vi "单次收发模式.vi"() -> ()   [LabVIEW 2017]
uses:
  <vilib>/Instr/_visa.llb/VISA Configure Serial Port (Instr).vi
  <vilib>/ptbypt/NI_PtbyPt.lvlib
panel:
  out "波形图表":cluster{dbl, dbl, dbl}(graph)
  out "Fz":dbl
  out "Fy":dbl
  out "Fx":dbl
  out "连接的字符串":string
  out "频率/Hz":dbl
  out "relative seconds":dbl caption="相对秒钟" format="%_19f"
  in  "置零":bool
  in  "停止":bool
  in  "传感器串口号":refnum<visa-resource-name>
  out "读取缓冲区":string
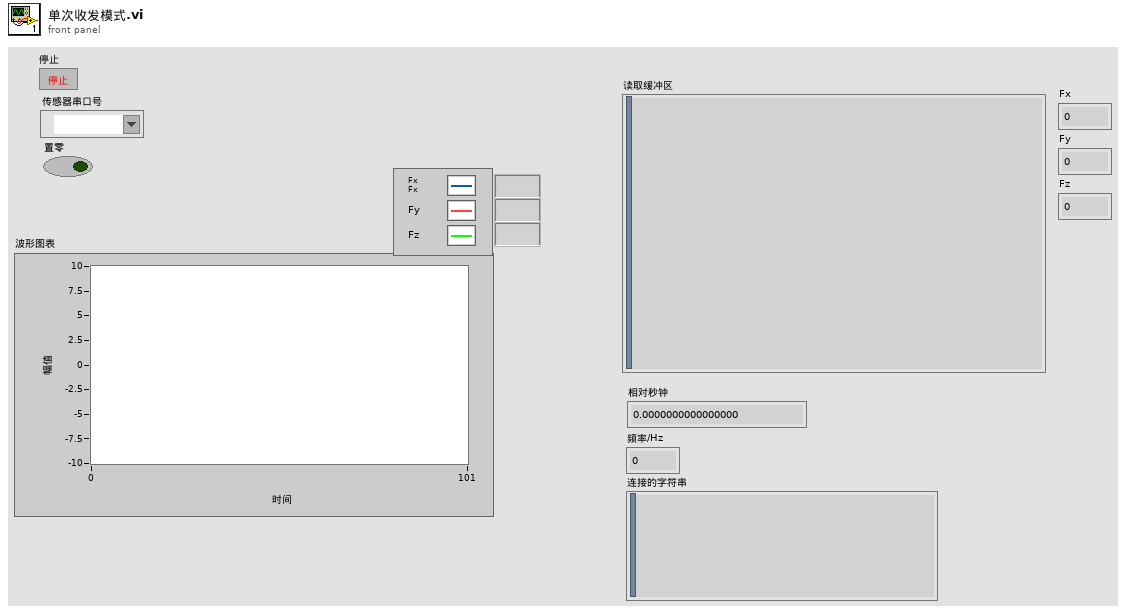
[diagram p1: front panel]
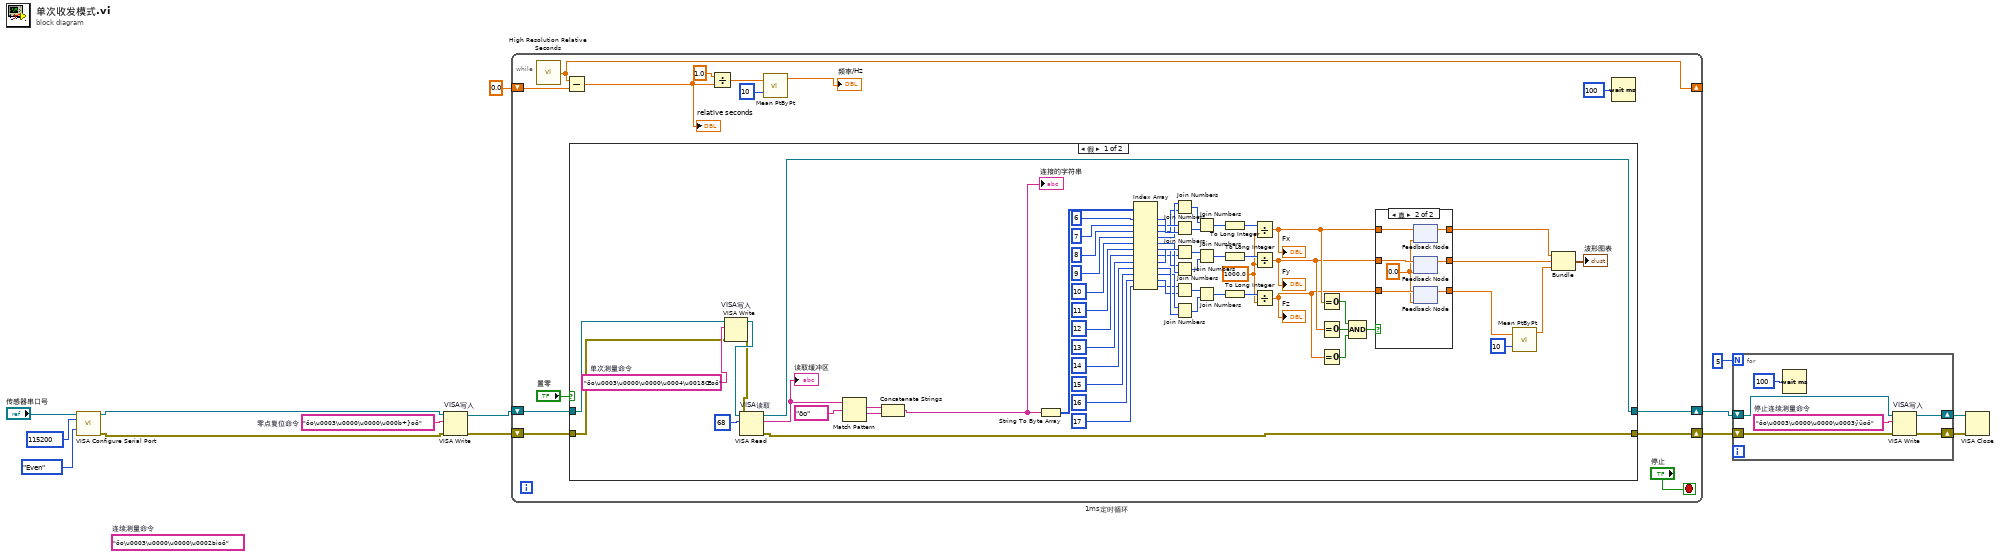
[diagram p0: block diagram]
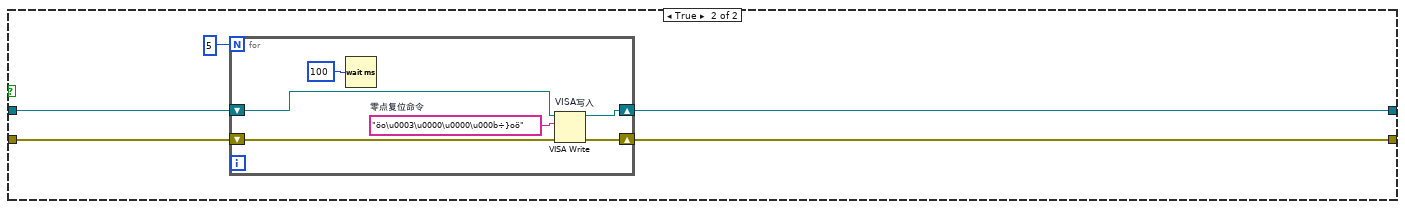
[diagram p3: hidden frame]
diagram:
  w2 = "öo\u0003\u0000\u0000\u000b÷}oö"  # 零点复位命令
  (unwired) "öo\u0003\u0000\u0000\u0002Þìoö"  # 连续测量命令
  n1 = call-poly "VISA Configure Serial Port"("VISA resource name"="传感器串口号", "baud rate (9600)"=u32 115200, "parity (0:none)"=enum16{"None", "Odd", "Even", "Mark", "Space"}."Even") -> ("VISA resource name out"=w12:refnum<visa-resource-name>, "error out"=w11:errorcluster)  [unwired: 11 in]
  n2 = VISA Write "VISA写入"(VISA resource name=w12, write buffer=w2, error in (no error)=w11) -> (VISA resource name out=w4:refnum<visa-resource-name>, error out=w3:errorcluster)  [unwired: 1 out]
  n3 = while "1ms定时循环" {
    shift-right: [w26] -> w9
    shift-left: w4 -> [w28]
    shift-right: [w25] -> w8
    shift-left: w3 -> [w27]
    shift-right: [w22] -> _
    shift-left: 0.0 ("relative seconds") -> [w21]
    stop <- "停止" stop-if-true
    n4 = call <vilib>:"High Resolution Relative Seconds.vi"() -> ("relative seconds"=w22:dbl)
    n5 = Subtract(x=w22, y=w21) -> (x-y=w20:dbl)
    "relative seconds" <- w20
    n6 = case shown="假" "置零" {
      tunnel: w28 -> [w33 w105]
      tunnel: w27 -> [w32 w107]
      tunnel: [w91 w104] -> w26
      tunnel: [w90 w106] -> w25
      frame False {
        w34 = "öo\u0003\u0000\u0000\u0004\u0018Œoö"  # 单次测量命令
        w59 = 1000.0
        n7 = VISA Write "VISA写入"(VISA resource name=w33, write buffer=w34, error in (no error)=w32) -> (VISA resource name out=w31:refnum<visa-resource-name>, error out=w30:errorcluster)  [unwired: 1 out]
        n8 = VISA Read "VISA读取"(VISA resource name=w31, byte count=u32 68 ("字节总数"), error in (no error)=w30) -> (VISA resource name out=w91:refnum<visa-resource-name>, read buffer=w89:string, error out=w90:errorcluster)  [unwired: 1 out]
        "读取缓冲区" <- w89
        n9 = Match Pattern(string=w89, regular expression="öo" ("正则表达式")) -> (match substring=w85:string, after substring=w84:string)  [unwired: 1 in, 2 out]
        n10 = Concatenate Strings(w85, w84) -> (w29:string)
        "连接的字符串" <- w29
        n11 = String To Byte Array(string=w29) -> (unsigned byte array=w87:u8[])
        n12 = Index Array(array=w87, index #1=6 ("索引"), index #2=7 ("索引"), index #3=8 ("索引"), index #4=9 ("索引"), index #5=10 ("索引"), index #6=11 ("索引"), index #7=12 ("索引"), index #8=13 ("索引"), index #9=14 ("索引"), index #10=15 ("索引"), index #11=16 ("索引"), index #12=17 ("索引")) -> (element #1=w83:u8, element #2=w82:u8, element #3=w80:u8, element #4=w81:u8, element #5=w73:u8, element #6=w72:u8, element #7=w71:u8, element #8=w74:u8, element #9=w66:u8, element #10=w65:u8, element #11=w64:u8, element #12=w63:u8)
        n13 = Join Numbers(hi=w81, lo=w80) -> ((hi.lo)=w78:u16)
        n14 = Join Numbers(hi=w82, lo=w83) -> ((hi.lo)=w79:u16)
        n15 = Join Numbers(hi=w74, lo=w71) -> ((hi.lo)=w76:u16)
        n16 = Join Numbers(hi=w72, lo=w73) -> ((hi.lo)=w75:u16)
        n17 = Join Numbers(hi=w63, lo=w64) -> ((hi.lo)=w67:u16)
        n18 = Join Numbers(hi=w65, lo=w66) -> ((hi.lo)=w68:u16)
        n19 = Join Numbers(hi=w78, lo=w79) -> ((hi.lo)=w77:u32)
        n20 = Join Numbers(hi=w76, lo=w75) -> ((hi.lo)=w70:u32)
        n21 = Join Numbers(hi=w67, lo=w68) -> ((hi.lo)=w69:u32)
        n22 = To Long Integer(number=w77) -> (32bit integer=w62:i32)
        n23 = To Long Integer(number=w70) -> (32bit integer=w60:i32)
        n24 = To Long Integer(number=w69) -> (32bit integer=w61:i32)
        n25 = Divide(x=w62, y=w59) -> (x/y=w42:dbl)
        "Fx" <- w42
        n26 = Divide(x=w60, y=w59) -> (x/y=w41:dbl)
        "Fy" <- w41
        n27 = Divide(x=w61, y=w59) -> (x/y=w40:dbl)
        "Fz" <- w40
        n28 = Equal To 0?(x=w42) -> (x = 0?=w46:bool)
        n29 = Equal To 0?(x=w41) -> (x = 0?=w45:bool)
        n30 = Equal To 0?(x=w40) -> (x = 0?=w44:bool)
        n31 = Compound Arithmetic op=AND ("复合运算")(w46, w45, w44) -> (w43:bool)
        n32 = case shown="真" w43 {
          tunnel: w42 -> [w95 w102]
          tunnel: w41 -> [w94 w100]
          tunnel: w40 -> [w93 w98]
          tunnel: [w95 w101] -> w39
          tunnel: [w94 w99] -> w38
          tunnel: [w93 w97] -> w37
          frame False {
          }
          frame True {
            w96 = 0.0
            n33 = feedback-in #1(w102) -> ()
            n34 = feedback #1(w96) -> (w101:dbl)
            n35 = feedback #2(w96) -> (w99:dbl)
            n36 = feedback-in #2(w100) -> ()
            n37 = feedback #3(w96) -> (w97:dbl)
            n38 = feedback-in #3(w98) -> ()
          }
        }
        n39 = call <vilib>:"Mean PtByPt.vi"("x"=w37, "sample length"=10) -> ("mean"=w35:dbl)  [unwired: 2 in, 1 out]
        n40 = Bundle(w39, w38, "mean"=w35) -> (→"波形图表":cluster{dbl, dbl, "mean":dbl})  [unwired: 1 in]
      }
      frame True {
        n41 = for {
          N: 5 -> [_]
          shift-right: [w111] -> w106
          shift-left: w107 -> [w112]
          shift-right: [w109] -> w104
          shift-left: w105 -> [w110]
          w113 = "öo\u0003\u0000\u0000\u000b÷}oö"  # 零点复位命令
          n42 = Wait (ms)(milliseconds to wait=u32 100 ("等待时间（毫秒）")) -> ()  [unwired: 1 out]
          n43 = VISA Write "VISA写入"(VISA resource name=w110, write buffer=w113, error in (no error)=w112) -> (VISA resource name out=w109:refnum<visa-resource-name>, error out=w111:errorcluster)  [unwired: 1 out]
        }
      }
    }
    n44 = Divide(x=1.0, y=w20) -> (x/y=w18:dbl)
    n45 = call <vilib>:"Mean PtByPt.vi"("x"=w18, "sample length"=10) -> ("mean"=→"频率/Hz":dbl)  [unwired: 2 in, 1 out]
    n46 = Wait (ms)(milliseconds to wait=u32 100 ("等待时间（毫秒）")) -> ()  [unwired: 1 out]
  }
  n47 = for {
    N: 5 -> [_]
    shift-right: [w116] -> w6
    shift-left: w9 -> [w119]
    shift-right: [w117] -> w7
    shift-left: w8 -> [w118]
    w115 = "öo\u0003\u0000\u0000\u0003ÿüoö"  # 停止连续测量命令
    n48 = Wait (ms)(milliseconds to wait=u32 100 ("等待时间（毫秒）")) -> ()  [unwired: 1 out]
    n49 = VISA Write "VISA写入"(VISA resource name=w119, write buffer=w115, error in (no error)=w118) -> (VISA resource name out=w116:refnum<visa-resource-name>, error out=w117:errorcluster)  [unwired: 1 out]
  }
  n50 = VISA Close(VISA resource name=w6, error in (no error)=w7) -> ()  [unwired: 1 out]
